vi "Threshold Max Image to ROIs.vi"(8 "Error In":errorcluster, 9 "Threshold":dbl, 11 "Image Refnum in":T2) -> (0 "Error Out":errorcluster, 2 "ROIs":T1[](array[typedef]) {"Contours"."Type" items=["No Selection", "Point", "Line", "Rectangle", "Oval", "Polygon", "Freehand Region", "Annulus", "Unused2", "Unused3", "Broken Line", "Freehand Line", "Rotated Rectangle"]})   [LabVIEW 2021, in "Image.lvlib"]
uses:
  Image.lvlib
  <vilib>/vision/Image Controls.llb/IMAQ Image.ctl
  <vilib>/vision/NI_Vision_Development_Module.lvlib
  Strings/Strings.lvlib
  Error/Error.lvlib
  Time/Time.lvlib
panel:
  out "CPU (s)":dbl
  out "#ROIs":i32
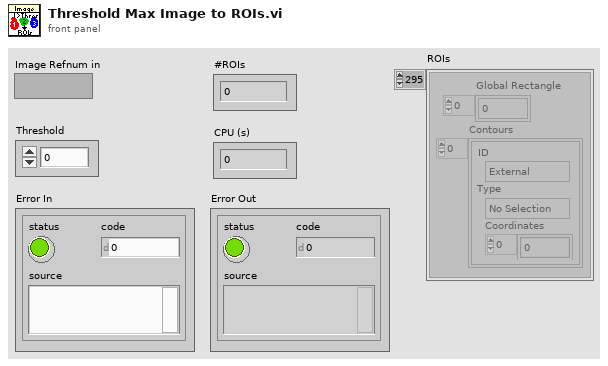
[diagram p1: front panel]
types:
  T1 = typedef "ROI Descriptor" = cluster{"Global Rectangle":i32[], "Contours":cluster{"ID":enum32{"External", "Internal"}, "Type":u32, "Coordinates":i32[]}[]}
  T2 = typedef "IMAQ Image.ctl" = refnum<image>
  T3 = enum32{"AutoM", "Close", "Dilate", "Erode", "Gradient", "Gradient in", "Gradient out", "HitMiss", "Open", "PClose", "POpen", "Thick", "Thin"}
  T4 = typedef "Particle Parameters" = i32
  T5 = cluster{"Measurement Parameter":T4, "Range Lower Value":dbl, "Range Upper Value":dbl, "Range":bool, "Measurement Type":bool}[]
  T6 = typedef "Image Type" = u32
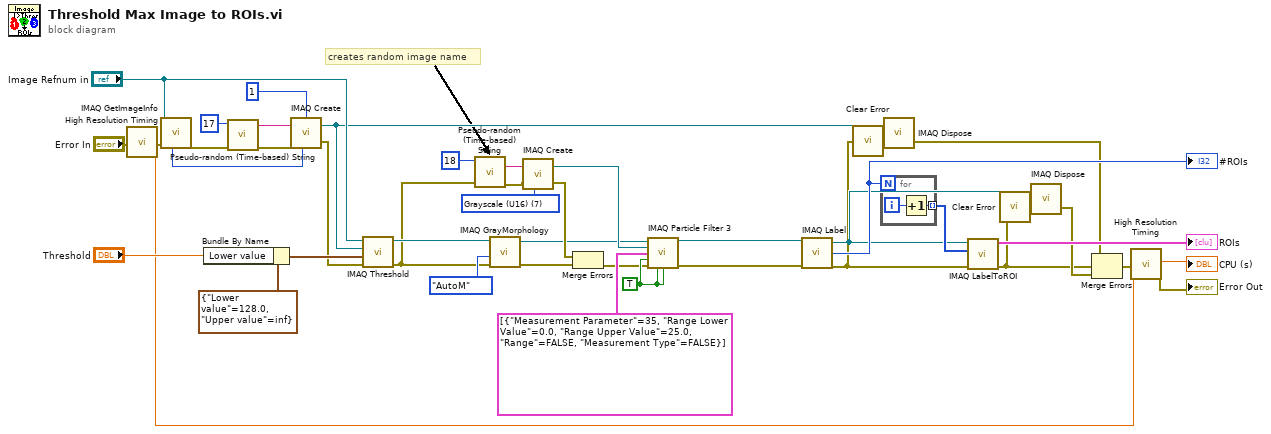
[diagram p0: block diagram]
diagram:
  w24 = TRUE ("Keep/Remove Particles (F)")
  w32 = T6 7 items=["Grayscale (U8)", "Grayscale (I16)", "Grayscale (SGL)", "Complex (CSG)", "RGB (U32)", "HSL (U32)", "RGB (U64)", "Grayscale (U16)"] ("Image Type")
  # "creates random image name"
  n1 = call "High Resolution Timing.vi"("Error In"="Error In") -> ("elapsed (relative) seconds"=w5:dbl, "Error Out"=w7:errorcluster)  [unwired: 16 in, 1 out]
  n2 = call "IMAQ GetImageInfo"("error in (no error)"=w7, "Image"="Image Refnum in") -> ("error out"=w17:errorcluster, "Image Type"=w33:T6)  [unwired: 2 in, 6 out]
  n3 = Bundle By Name(cluster=cluster{"Lower value":sgl, "Upper value":sgl} {"Lower value"=128.0, "Upper value"=inf} ("Range"), "Lower value"="Threshold") -> (w40:cluster{"Lower value":sgl, "Upper value":sgl})
  n4 = call "Pseudo-random (Time-based) String.vi"("Error In"=w17, "Length (10)"=u32 17) -> ("Error Out"=w16:errorcluster, "result string"=w18:string)  [unwired: 8 in]
  n5 = call "IMAQ Create"("Border Size"=1, "Image Name"=w18, "Image Type"=w33, "error in (no error)"=w16) -> ("New Image"=w31:T2, "error out"=w38:errorcluster)  [unwired: 1 in]
  n6 = call "IMAQ Threshold"("error in (no error)"=w38, "Range"=w40, "Image Dst"=w31, "Image Src"="Image Refnum in") -> ("error out"=w15:errorcluster, "Image Dst Out"=w22:T2)  [unwired: 6 in]
  n7 = call "Pseudo-random (Time-based) String.vi"("Error In"=w15, "Length (10)"=u32 18) -> ("Error Out"=w14:errorcluster, "result string"=w13:string)  [unwired: 8 in]
  n8 = call "IMAQ GrayMorphology"("error in (no error)"=w15, "Operation"=T3."AutoM", "Image Src"=w22) -> ("error out"=w20:errorcluster, "Image Dst Out"=w23:T2)  [unwired: 7 in]
  n9 = call "IMAQ Create"("Image Name"=w13, "Image Type"=w32, "error in (no error)"=w14) -> ("New Image"=w29:T2, "error out"=w27:errorcluster)  [unwired: 2 in]
  n10 = Merge Errors(w27, w20) -> (w21:errorcluster)
  n11 = call "IMAQ Particle Filter 3"("Image Src"=w23, "Image Dst"=w29, "Selection Values"=T5 [{"Measurement Parameter"=35, "Range Lower Value"=0.0, "Range Upper Value"=25.0, "Range"=FALSE, "Measurement Type"=FALSE}], "Keep/Remove Particles (F)"=w24, "error in (no error)"=w21, "Reject Border? (F)"=w24, "Fill Holes? (F)"=w24) -> ("Image Dst Out"=w28:T2, "error out"=w26:errorcluster)  [unwired: 6 in, 1 out]
  n12 = call "IMAQ Label"("error in (no error)"=w26, "Image Src"=w28) -> ("error out"=w30:errorcluster, "Number of Particles"=w44:i32, "Image Dst Out"=w37:T2)  [unwired: 2 in]
  "#ROIs" <- w44
  n13 = call "Clear Error.vi"("Error In"=w30) -> ("no Error Out"=w3:errorcluster)  [unwired: 8 in]
  n14 = for {
    N: w44 -> [_]
    tunnel: [w45] -> w43 mode=indexing
    i -> [w46]
    n15 = Increment(x=w46) -> (x+1=w45:i32)
  }
  n16 = call "IMAQ Dispose"("Image"=w31, "error in (no error)"=w3) -> ("error out"=w2:errorcluster)  [unwired: 4 in]
  n17 = call "IMAQ LabelToROI"("error in (no error)"=w30, "Labels In"=w43, "Image"=w37) -> ("error out"=w8:errorcluster, "ROIs"=→"ROIs":T1[])  [unwired: 5 in, 2 out]
  n18 = call "Clear Error.vi"("Error In"=w8) -> ("no Error Out"=w10:errorcluster)  [unwired: 8 in]
  n19 = call "IMAQ Dispose"("Image"=w37, "error in (no error)"=w10) -> ("error out"=w36:errorcluster)  [unwired: 4 in]
  n20 = Merge Errors(w2, w8, w36) -> (w9:errorcluster)
  n21 = call "High Resolution Timing.vi"("relative seconds (NaN)"=w5, "Error In"=w9) -> ("elapsed (relative) seconds"=→"CPU (s)":dbl, "Error Out"=→"Error Out":errorcluster)  [unwired: 15 in, 1 out]
